vi "Write write enable.vi"(8 "error in (no error)":errorcluster, 10 "write enable":bool, 11 "Master CR in":refnum<class "WebSocket Client CR.lvclass">) -> (0 "error out":errorcluster, 3 "Master CR out":refnum<class "WebSocket Client CR.lvclass">)   [LabVIEW 2021, in "WebSockets.lvlib" / "WebSocket Client CR.lvclass"]
uses:
  WebSocket Client CR.lvclass
  WebSocket Client CR.lvclass/WebSocket Client CR.ctl
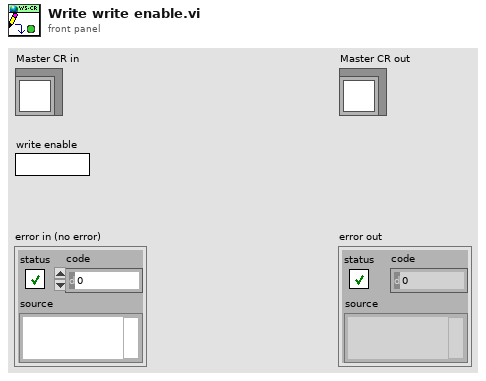
[diagram p1: front panel]
types:
  T1 = typedef "WebSockets.lvlib/WebSocket Client CR.lvclass/Master CR state.ctl" = cluster{"state":T2, "enable":bool, "write enable":bool, "connect":bool, "errors":i32, "Run":bool, "Write":bool, "Stop":bool}
  T2 = typedef "WebSockets.lvlib/WebSocket Client CR.lvclass/CR_Core_State.ctl" = enum8{"initialization", "redefine", "standby", "ping", "connect", "wait to reconnect", "wait to reset timeout", "configure", "requests", "close connection", "stop"}
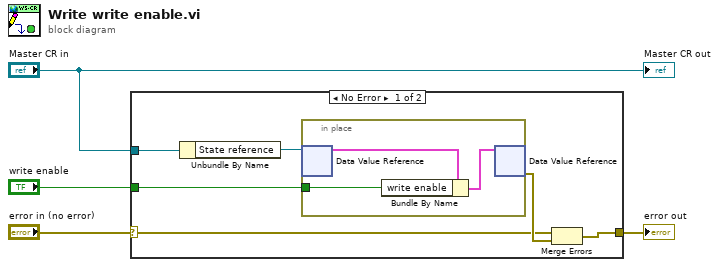
[diagram p0: block diagram]
diagram:
  n1 = case shown="No Error" "error in (no error)" {
    selector: "error in (no error)" -> [w5 w14]
    tunnel: [w8 w14] -> w3
    tunnel: "Master CR in" -> [w6 _]
    tunnel: "write enable" -> [w7 _]
    frame No Error {
      n2 = Unbundle By Name(w6) -> ("State reference"=w10:refnum<data-value>)
      n3 = in-place {
        in-place-border: w7 -> [w11]
        n4 = in-place-dvr #1(w10) -> (w13:T1)  [unwired: 1 out]
        n5 = Bundle By Name(cluster=w13, "write enable"=w11) -> (w12:T1)
        n6 = in-place-dvr #1(w12) -> (w9:errorcluster)  [unwired: 1 out]
      }
      n7 = Merge Errors(w5, w9) -> (w8:errorcluster)
    }
    frame Error {
    }
  }
  "error out" <- w3
  "Master CR out" <- "Master CR in"
